vi "Untitled 1 (SubVI).vi"(9 "X":dbl, 10 "Y":dbl) -> (1 "Roll":dbl, 2 "Hover":bool, 3 "Pitch":dbl)   [LabVIEW 2014]
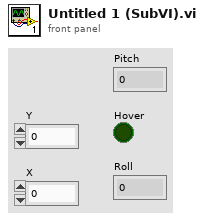
[diagram p1: front panel]
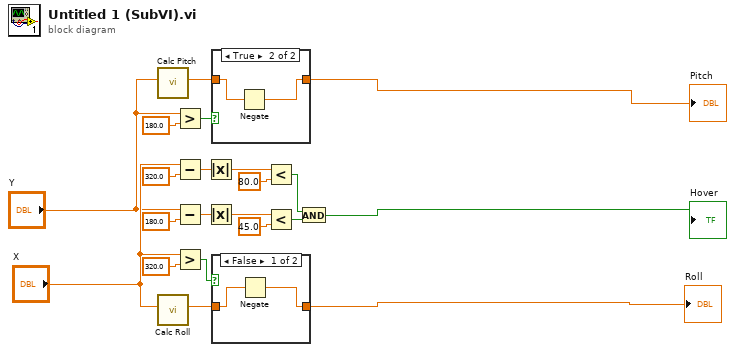
[diagram p0: block diagram]
diagram:
  n1 = call "Calc Pitch.vi"("Position"="Y") -> ("Pitch"=w8:dbl)  [unwired: 10 in]
  n2 = call "Calc Roll.vi"("Position"="X") -> ("Roll"=w9:dbl)  [unwired: 10 in]
  n3 = Greater?(x="Y", y=180.0) -> (0:w5:bool)
  n4 = Subtract(x="X", y=320.0) -> (x-y=w15:dbl)
  n5 = Subtract(x="Y", y=180.0) -> (x-y=w10:dbl)
  n6 = Greater?(x="X", y=320.0) -> (0:w7:bool)
  n7 = Absolute Value(x=w15) -> (abs(x)=w17:dbl)
  n8 = Absolute Value(x=w10) -> (abs(x)=w13:dbl)
  n9 = case shown="True" w5 {
    tunnel: w8 -> [w22 w24]
    tunnel: [w22 w23] -> w3
    frame False {
    }
    frame True {
      n10 = Negate(x=w24) -> (-x=w23:dbl)
    }
  }
  "Pitch" <- w3
  n11 = case shown="False" w7 {
    tunnel: w9 -> [w26 w27]
    tunnel: [w25 w27] -> w2
    frame False {
      n12 = Negate(x=w26) -> (-x=w25:dbl)
    }
    frame True {
    }
  }
  "Roll" <- w2
  n13 = Less?(x=w17, y=80.0) -> (x < y?=w20:bool)
  n14 = Less?(x=w13, y=45.0) -> (x < y?=w21:bool)
  n15 = And(x=w20, y=w21) -> (x .and. y?=→"Hover":bool)
